vi "Write Step rate.vi"(10 "Step rate":u32=1000, 11 "Dummy Job in":refnum<class "Dummy Job.lvclass">) -> (3 "Dummy Job out":refnum<class "Dummy Job.lvclass">)   [LabVIEW 2014, in "Dummy Job.lvclass"]
uses:
  Dummy Job.lvclass
  Dummy Job.lvclass/Dummy Job.ctl
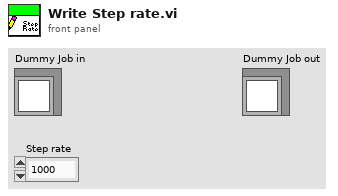
[diagram p1: front panel]
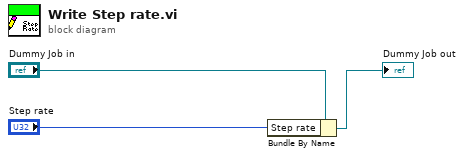
[diagram p0: block diagram]
diagram:
  n1 = Bundle By Name(cluster="Dummy Job in", "Step rate"="Step rate") -> (→"Dummy Job out":refnum<class "Dummy Job.lvclass">)
